vi "Read Database.vi"(8 "error in (no error)":errorcluster) -> (0 "error out":errorcluster, 3 "data":i32[](array[numeric]))   [LabVIEW 2017]
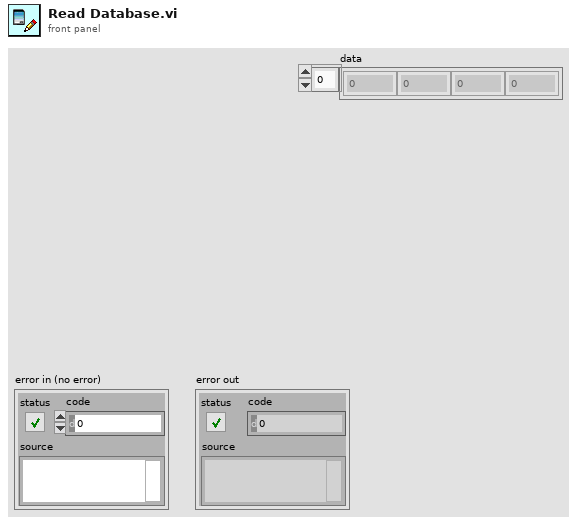
[diagram p1: front panel]
types:
  T1 = enum16{"open", "replace", "create", "open or create", "replace or create", "replace or create with confirmation"}
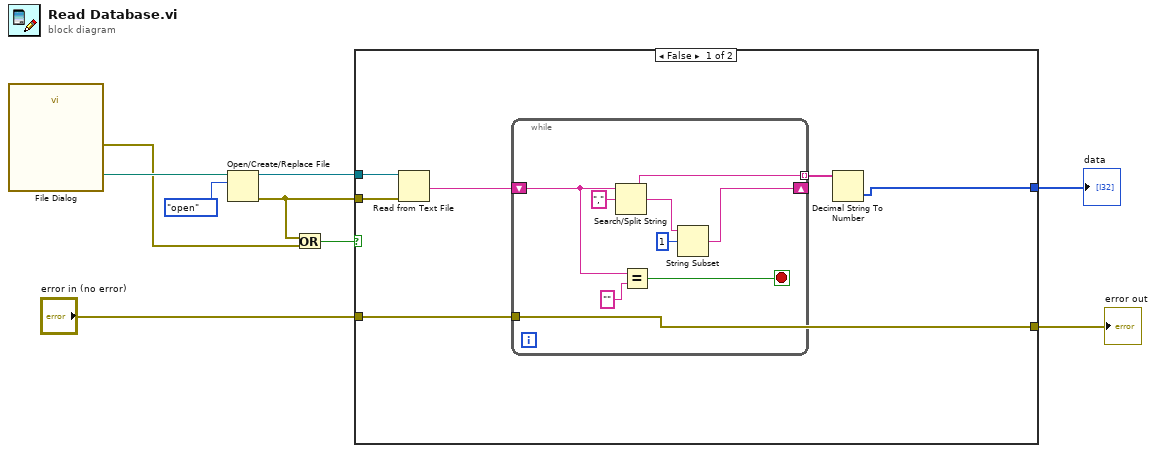
[diagram p0: block diagram]
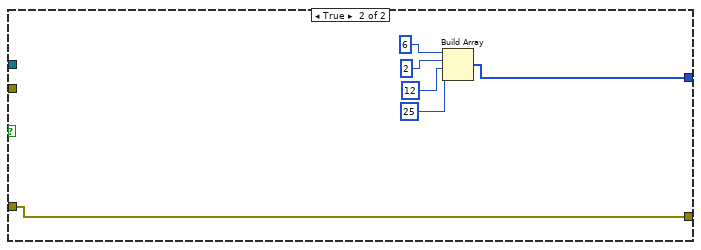
[diagram p2: hidden frame]
diagram:
  n1 = call "File Dialog"() -> ("selected path"=w7:path, "error out"=w2:errorcluster)  [unwired: 12 in, 2 out]
  n2 = Open/Create/Replace File(file path (use dialog)=w7, operation (0:open)=T1."open") -> (refnum out=w9:refnum<file>, error out=w3:errorcluster)  [unwired: 4 in, 1 out]
  n3 = Or(x=w3, y=w2) -> (x .or. y?=w1:bool)
  n4 = case shown="False" w1 {
    tunnel: w9 -> [w16 _]
    tunnel: w3 -> [w15 _]
    tunnel: "error in (no error)" -> [w13 w26]
    tunnel: [w11 w27] -> w5
    tunnel: [w10 w26] -> w4
    frame False {
      n5 = Read from Text File(file (use dialog)=w16, error in=w15) -> (text=w14:string)  [unwired: 2 in, 3 out]
      n6 = while {
        tunnel: [w24] -> w12 mode=indexing
        shift-right: [w18] -> _
        shift-left: w14 -> [w23]
        tunnel: w13 -> [w17]
        tunnel: [w17] -> w10
        stop <- w21 stop-if-true
        n7 = Search/Split String(string=w23, search string/char (-)=",") -> (substring before match=w24:string, match + rest of string=w19:string)  [unwired: 1 in, 1 out]
        n8 = Equal?(x=w23, y="") -> (x = y?=w21:bool)
        n9 = String Subset(string=w19, offset (0)=1) -> (substring=w18:string)  [unwired: 1 in]
      }
      n10 = Decimal String To Number(string=w12) -> (number=w11:i32[])  [unwired: 2 in, 1 out]
    }
    frame True {
      n11 = Build Array(6, 2, 12, 25) -> (w27:i32[])
    }
  }
  "data" <- w5
  "error out" <- w4
